vi "Execute.vi"(1 "Numeric":dbl, 4 "Position":i32, 6 "Assembly Type":string, 8 "error in (no error)":errorcluster, 9 "Workspace":T1, 10 "Control In":T2={"I-O.lvclass"=refnum, "Gantry"=refnum, "Dispenser"="COM1"}, 11 "Secure Syringe in":refnum<class "SecureRelease Syringe.lvclass">) -> (0 "error out":errorcluster, 2 "Control Out":T2={"I-O.lvclass"=refnum, "Gantry"=refnum, "Dispenser"="COM1"}, 3 "Secure Syringe out":refnum<class "SecureRelease Syringe.lvclass">)   [LabVIEW 2021, in "SecureRelease Syringe.lvclass"]
uses:
  SecureRelease Syringe.lvclass
  Controller/Controllers.ctl
  Controller/I-O/I-O.lvclass
  C:/Program Files (x86)/Aerotech/A3200/LabVIEW/2010/Bin/Aerotech.A3200.dll
  Program Files (x86)/Aerotech/A3200/LabVIEW/2010/Bin/Aerotech.A3200.dll
  Workspace/Workspace.ctl
  SecureRelease Syringe.lvclass/SecureRelease Syringe.ctl
  Controller/Motion/Motion.lvclass
  Dispense/Dispense.lvclass
  Controller/Motion/A3200/A3200.lvclass
  Controller/Dispenser/Dispenser.lvclass
  Controller/Controller.lvclass
  Workspace/Fixture.lvclass
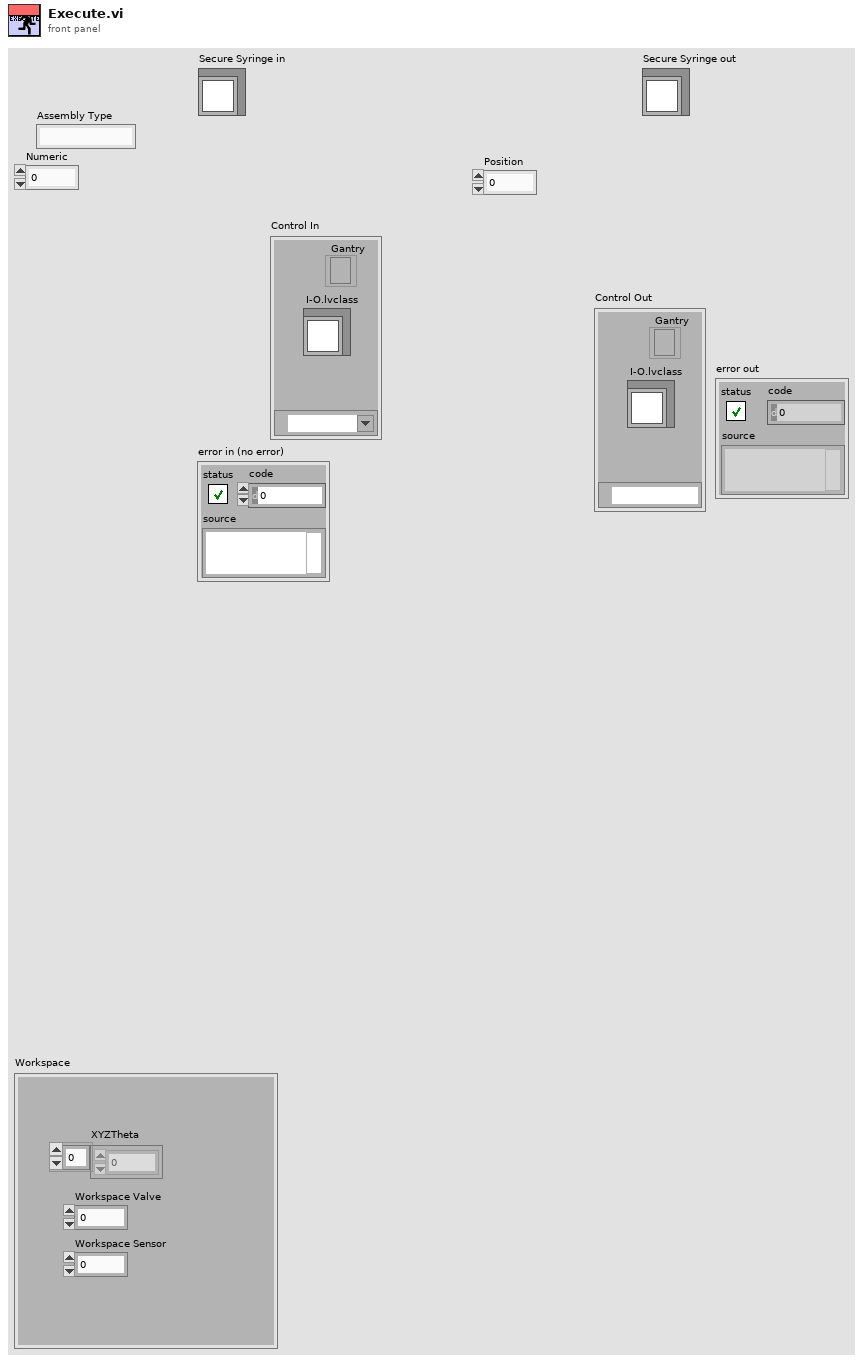
[diagram p1: front panel]
types:
  T1 = typedef "Fixture.lvclass/Workspace.ctl" = cluster{"XYZTheta":dbl[], "Workspace Valve":i32, "Workspace Sensor":i32}
  T2 = typedef "Controller.lvclass/Controllers.ctl" = cluster{"I-O.lvclass":refnum<class "I-O.lvclass">, "Gantry":refnum<k24>, "Dispenser":refnum<visa-resource-name>}
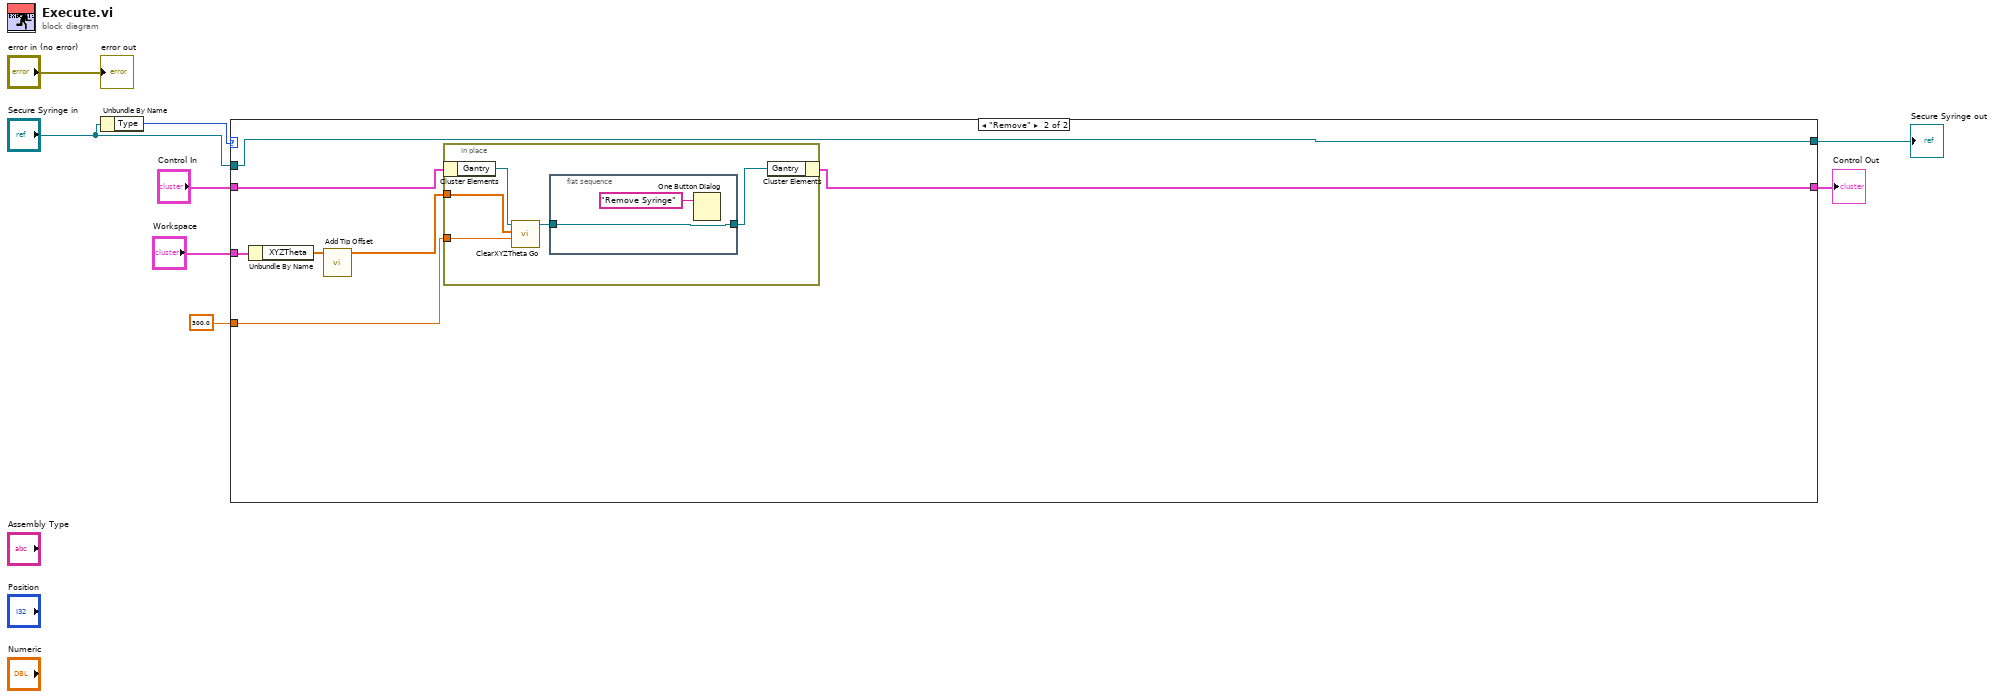
[diagram p0: block diagram]
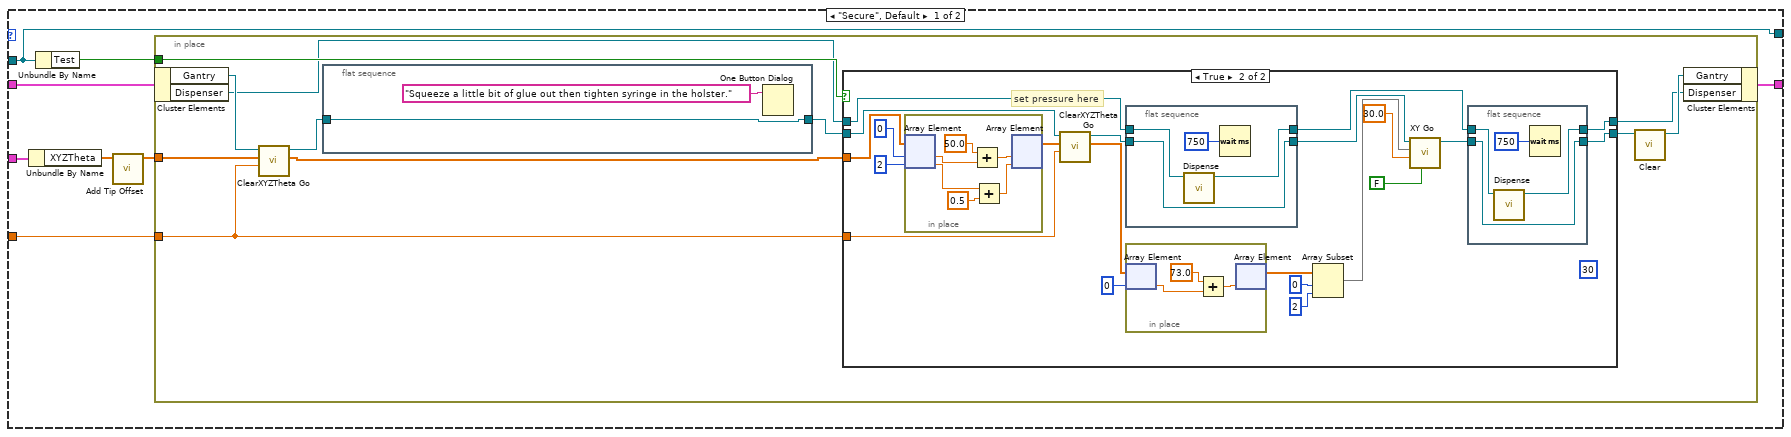
[diagram p2: hidden frame]
diagram:
  n1 = Unbundle By Name("Secure Syringe in") -> ("Type"=w2:enum16{"Secure", "Remove"})
  n2 = case shown="\"Remove\"" w2 {
    tunnel: "Workspace" -> [w16 w73]
    tunnel: "Secure Syringe in" -> [w12 w74]
    tunnel: [w12 w74] -> w6
    tunnel: "Control In" -> [w15 w75]
    tunnel: [w14 w76] -> w4
    tunnel: 300.0 ("Speed") -> [w9 w70]
    frame "Secure", Default {
      n3 = Unbundle By Name(w16) -> ("XYZTheta"=w11:dbl[])
      n4 = Unbundle By Name(w12) -> ("Test"=w13:bool)
      n5 = call "Add Tip Offset.vi"("XYZTheta"=w11) -> ("XYZTheta"=w10:dbl[])  [unwired: 10 in]
      n6 = in-place {
        in-place-border: w10 -> [w26]
        in-place-border: w13 -> [w20]
        in-place-border: w9 -> [w17]
        n7 = in-place-cluster #1(w15) -> ("Gantry"=w27:refnum<k24>, "Dispenser"=w19:refnum<visa-resource-name>)
        n8 = call "ClearXYZTheta Go.vi"("Speed"=w17, "XYZTheta In"=w26, "Gantry In"=w27) -> ("XYZTheta Out"=w21:dbl[], "Gantry Out"=w25:refnum<k24>)  [unwired: 6 in, 1 out]
        n9 = flat-sequence {
          tunnel: [w68] -> w23
          tunnel: w25 -> [w68]
          frame #0 {
            n10 = One Button Dialog(message="Squeeze a little bit of glue out then tighten syringe in the holster.") -> ()  [unwired: 1 in, 1 out]
          }
        }
        n11 = case shown="True" w20 {
          tunnel: w23 -> [w29 w50]
          tunnel: [w29 w42] -> w22
          tunnel: w21 -> [_ w49]
          tunnel: w19 -> [w28 w32]
          tunnel: [w28 w40] -> w18
          tunnel: w17 -> [_ w30]
          frame False {
          }
          frame True {
            (unwired) i16 30 ("Pressure")
            # "set pressure here"
            n12 = in-place {
              n13 = in-place-array #2(w49, 0, 2) -> (w67:dbl, w65:dbl)
              n14 = Add(x=50.0, y=w67) -> (x+y=w62:dbl)
              n15 = Add(x=w65, y=0.5) -> (x+y=w63:dbl)
              n16 = in-place-array #2(w62, w63) -> (w46:dbl[])  [unwired: 2 out]
            }
            n17 = call "ClearXYZTheta Go.vi"("Speed"=w30, "XYZTheta In"=w46, "Gantry In"=w50) -> ("XYZTheta Out"=w45:dbl[], "Gantry Out"=w43:refnum<k24>)  [unwired: 6 in, 1 out]
            n18 = flat-sequence {
              tunnel: [w58] -> w34
              tunnel: w43 -> [w58]
              tunnel: w32 -> [w55]
              tunnel: [w56] -> w41
              frame #0 {
                n19 = call "Dispense.vi"("Dispenser In"=w55) -> ("Dispenser Out"=w56:refnum<visa-resource-name>)  [unwired: 9 in, 1 out]
                n20 = Wait (ms)(milliseconds to wait=u32 750) -> ()  [unwired: 1 out]
              }
            }
            n21 = in-place {
              n22 = in-place-array #3(w45, 0) -> (w61:dbl)
              n23 = Add(x=73.0, y=w61) -> (x+y=w59:dbl)
              n24 = in-place-array #3(w59) -> (w39:dbl[])  [unwired: 1 out]
            }
            n25 = Array Subset(array=w39, index=0, length=2) -> (w36:dbl[])
            n26 = call "XY Go.vi"("return immediately"=FALSE, "Speed"=30.0, "XY In"=w36, "Gantry In"=w34) -> ("Gantry Out"=w33:refnum<k24>)  [unwired: 5 in, 2 out]
            n27 = flat-sequence {
              tunnel: [w54] -> w42
              tunnel: w33 -> [w54]
              tunnel: w41 -> [w51]
              tunnel: [w52] -> w40
              frame #0 {
                n28 = call "Dispense.vi"("Dispenser In"=w51) -> ("Dispenser Out"=w52:refnum<visa-resource-name>)  [unwired: 9 in, 1 out]
                n29 = Wait (ms)(milliseconds to wait=u32 750) -> ()  [unwired: 1 out]
              }
            }
          }
        }
        n30 = call "Clear.vi"("Gantry In"=w22) -> ("Gantry Out"=w24:refnum<k24>)  [unwired: 9 in, 1 out]
        n31 = in-place-cluster #1("Gantry"=w24, "Dispenser"=w18) -> (w14:T2)
      }
    }
    frame "Remove" {
      n32 = Unbundle By Name(w73) -> ("XYZTheta"=w71:dbl[])
      n33 = call "Add Tip Offset.vi"("XYZTheta"=w71) -> ("XYZTheta"=w72:dbl[])  [unwired: 10 in]
      n34 = in-place {
        in-place-border: w72 -> [w78]
        in-place-border: w70 -> [w77]
        n35 = in-place-cluster #4(w75) -> ("Gantry"=w81:refnum<k24>)
        n36 = call "ClearXYZTheta Go.vi"("Speed"=w77, "XYZTheta In"=w78, "Gantry In"=w81) -> ("Gantry Out"=w80:refnum<k24>)  [unwired: 6 in, 2 out]
        n37 = flat-sequence {
          tunnel: w80 -> [w83]
          tunnel: [w83] -> w79
          frame #0 {
            n38 = One Button Dialog(message="Remove Syringe") -> ()  [unwired: 1 in, 1 out]
          }
        }
        n39 = in-place-cluster #4("Gantry"=w79) -> (w76:T2)
      }
    }
  }
  "Secure Syringe out" <- w6
  "Control Out" <- w4
  "error out" <- "error in (no error)"
